vi "Virtual Assistant.vi"() -> ()   [LabVIEW 2018]
uses:
  Documents/Control 2.ctl
panel:
  out "Information":string
  out "Information":string
  in  "IMAGE File Path":path
  in  "?":bool
  in  "IMAGE File Path":path
  in  "?":bool
  in  "AUDIO File Path":path
  out "Information":string
  in  "?":bool
  in  "Enter object name":string
  # "This simulation is limited by various constraints. We require NI vision module/library for object recognization . So we have assumed that the output from the object recognization process is a string and designed the further simulation. Also we faved similar problems with audio processing and implemented the same methodology. \nWe hope these problems can be overcome provided we have access to full version of NI labview.\nBecause of those constraints , the search via audio file and image file will not work.Only Search via text will work properly.\nPlease simulate the seach via text using the following keywords. they are - uno,mega,rio,rpi,nodem cu,relay,ultrasonic,optocoupler,servomotor,dc-motor,stepper-motor,resistor,capacitor,inductor,microcontroller,battery,microprocessor,diode,transistor,fuse.\nBecause we have given the database with these details only."
  # "Ideal case"
  # "Ideal case"
  # "Working Case"
  # "SEARCH via TEXT"
  # "SEARCH via AUDIO FILE"
  # "SEARCH via IMAGE FILE"
  # "NOTE: All the information is given in the Document for the simulation of this project. Please Read the document first."
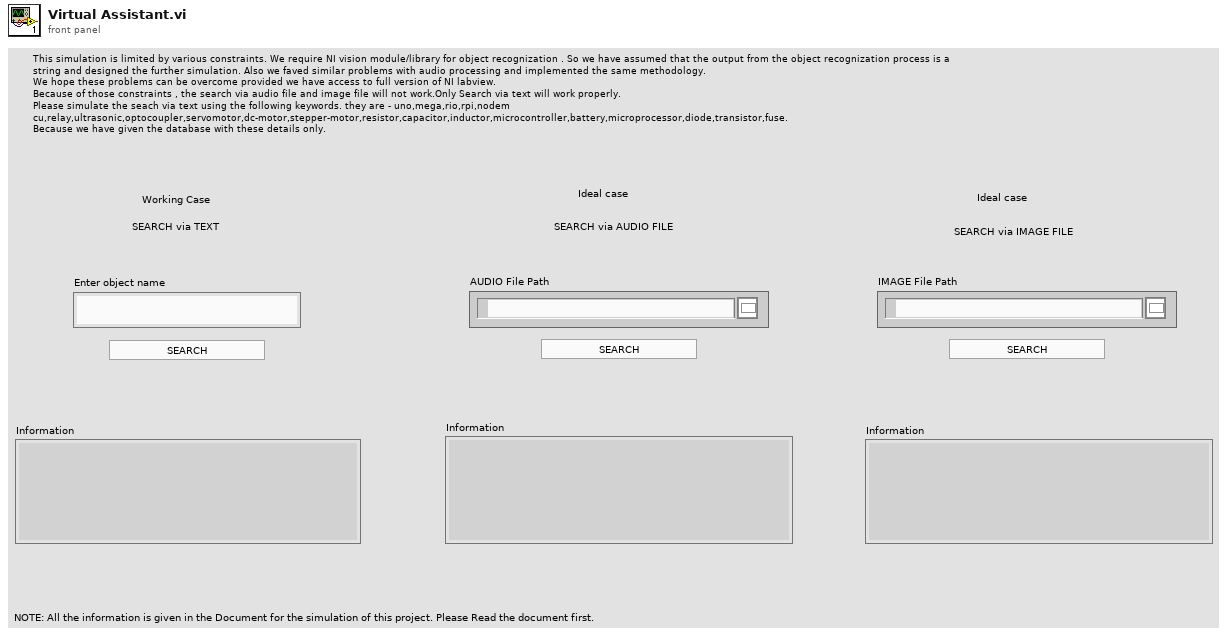
[diagram p1: front panel]
types:
  T1 = typedef "Control 2.ctl" = enum16{"Text", "Image", "Audio"}
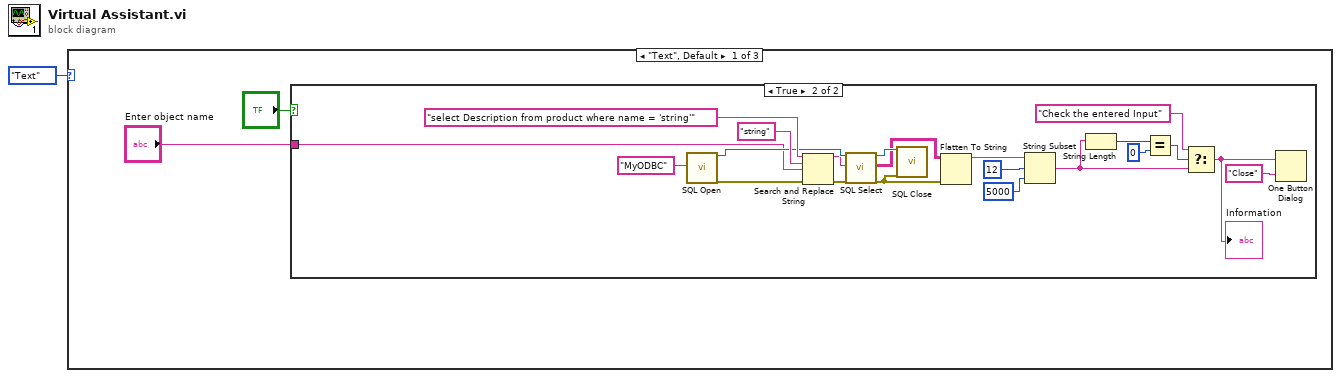
[diagram p0: block diagram]
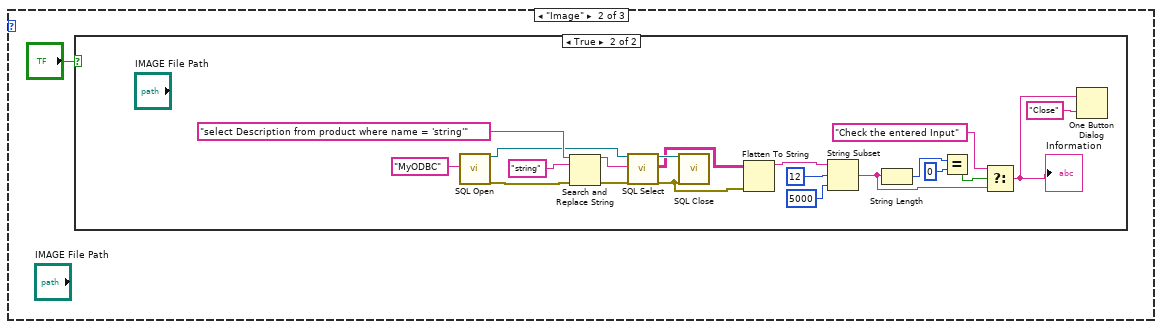
[diagram p3: hidden frame]
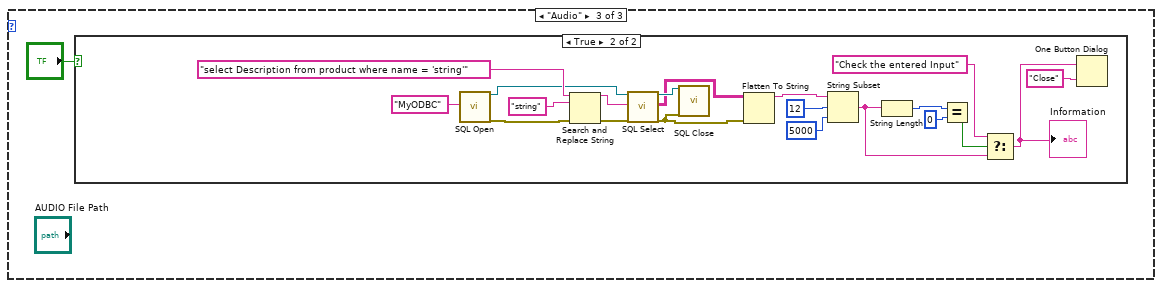
[diagram p5: hidden frame]
diagram:
  n1 = case shown="\"Text\", Default" Control_2."Text" {
    frame "Text", Default {
      n2 = case shown="True" "?" {
        tunnel: "Enter object name" -> [_ w6]
        frame False {
        }
        frame True {
          n3 = call <vilib>:"SQL Open.vi"("ConnectionString In"="MyODBC") -> ("Connection Out"=w21:refnum<k7>, "Error out"=w7:errorcluster)  [unwired: 17 in]
          n4 = Search and Replace String(input string="select Description from product where name = 'string'", search string="string", replace string=w6, error in=w7) -> (result string=w20:string, error out=w18:errorcluster)  [unwired: 4 in, 2 out]
          n5 = call <vilib>:"SQL Select.vi"("Connection In"=w21, "SQL Query"=w20, "Error in (no error)"=w18) -> ("Connection Out"=w19:refnum<k7>, "Data"=w17:string[][], "Error out"=w16:errorcluster)  [unwired: 14 in]
          n6 = call <vilib>:"SQL Close.vi"("Connection In"=w19, "Error in (no error)"=w16) -> ()  [unwired: 17 in, 1 out]
          n7 = Flatten To String(anything=w17, error in (no error)=w16) -> (data string=w13:string)  [unwired: 2 in, 2 out]
          n8 = String Subset(string=w13, offset (0)=12, length (rest)=5000 ("length (rest)")) -> (substring=w9:string)
          n9 = String Length(string=w9) -> (length=w12:i32)
          n10 = Equal?(x=w12, y=0) -> (x = y?=w10:bool)
          n11 = Select(t="Check the entered Input", s=w10, f=w9) -> (s? t:f=w5:string)
          "Information" <- w5
          n12 = One Button Dialog(message=w5, button name ("OK")="Close") -> ()  [unwired: 1 out]
        }
      }
    }
    frame "Image" {
      n13 = case shown="True" "?" {
        frame False {
        }
        frame True {
          n14 = call <vilib>:"SQL Open.vi"("ConnectionString In"="MyODBC") -> ("Connection Out"=w42:refnum<k7>, "Error out"=w28:errorcluster)  [unwired: 17 in]
          n15 = Search and Replace String(input string="select Description from product where name = 'string'", search string="string", error in=w28) -> (result string=w41:string, error out=w39:errorcluster)  [unwired: 5 in, 2 out]
          n16 = call <vilib>:"SQL Select.vi"("Connection In"=w42, "SQL Query"=w41, "Error in (no error)"=w39) -> ("Connection Out"=w40:refnum<k7>, "Data"=w38:string[][], "Error out"=w37:errorcluster)  [unwired: 14 in]
          n17 = call <vilib>:"SQL Close.vi"("Connection In"=w40, "Error in (no error)"=w37) -> ()  [unwired: 17 in, 1 out]
          n18 = Flatten To String(anything=w38, error in (no error)=w37) -> (data string=w34:string)  [unwired: 2 in, 2 out]
          n19 = String Subset(string=w34, offset (0)=12, length (rest)=5000 ("length (rest)")) -> (substring=w30:string)
          n20 = String Length(string=w30) -> (length=w33:i32)
          n21 = Equal?(x=w33, y=0) -> (x = y?=w31:bool)
          n22 = Select(t="Check the entered Input", s=w31, f=w30) -> (s? t:f=w26:string)
          "Information" <- w26
          n23 = One Button Dialog(message=w26, button name ("OK")="Close") -> ()  [unwired: 1 out]
        }
      }
    }
    frame "Audio" {
      n24 = case shown="True" "?" {
        frame False {
        }
        frame True {
          n25 = call <vilib>:"SQL Open.vi"("ConnectionString In"="MyODBC") -> ("Connection Out"=w63:refnum<k7>, "Error out"=w49:errorcluster)  [unwired: 17 in]
          n26 = Search and Replace String(input string="select Description from product where name = 'string'", search string="string", error in=w49) -> (result string=w62:string, error out=w60:errorcluster)  [unwired: 5 in, 2 out]
          n27 = call <vilib>:"SQL Select.vi"("Connection In"=w63, "SQL Query"=w62, "Error in (no error)"=w60) -> ("Connection Out"=w61:refnum<k7>, "Data"=w59:string[][], "Error out"=w58:errorcluster)  [unwired: 14 in]
          n28 = call <vilib>:"SQL Close.vi"("Connection In"=w61, "Error in (no error)"=w58) -> ()  [unwired: 17 in, 1 out]
          n29 = Flatten To String(anything=w59, error in (no error)=w58) -> (data string=w55:string)  [unwired: 2 in, 2 out]
          n30 = String Subset(string=w55, offset (0)=12, length (rest)=5000 ("length (rest)")) -> (substring=w51:string)
          n31 = String Length(string=w51) -> (length=w54:i32)
          n32 = Equal?(x=w54, y=0) -> (x = y?=w52:bool)
          n33 = Select(t="Check the entered Input", s=w52, f=w51) -> (s? t:f=w47:string)
          "Information" <- w47
          n34 = One Button Dialog(message=w47, button name ("OK")="Close") -> ()  [unwired: 1 out]
        }
      }
    }
  }
